vi "LMS_GetLPFBWRange.vi"(8 "error in (no error)":errorcluster, 10 "dir_tx":u8, 11 "device_In":i64) -> (0 "error out":errorcluster, 1 "range":cluster{"min":dbl, "max":dbl, "step":dbl}, 3 "device_Out":i64)   [LabVIEW 2018, in "LMS_LV_Drv.lvlib"]
uses:
  LMS_LV_Drv.lvlib
  C:/Program Files/PothosSDR/bin/LimeSuite.dll
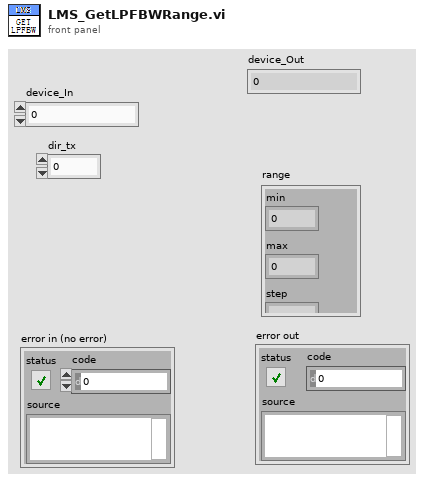
[diagram p1: front panel]
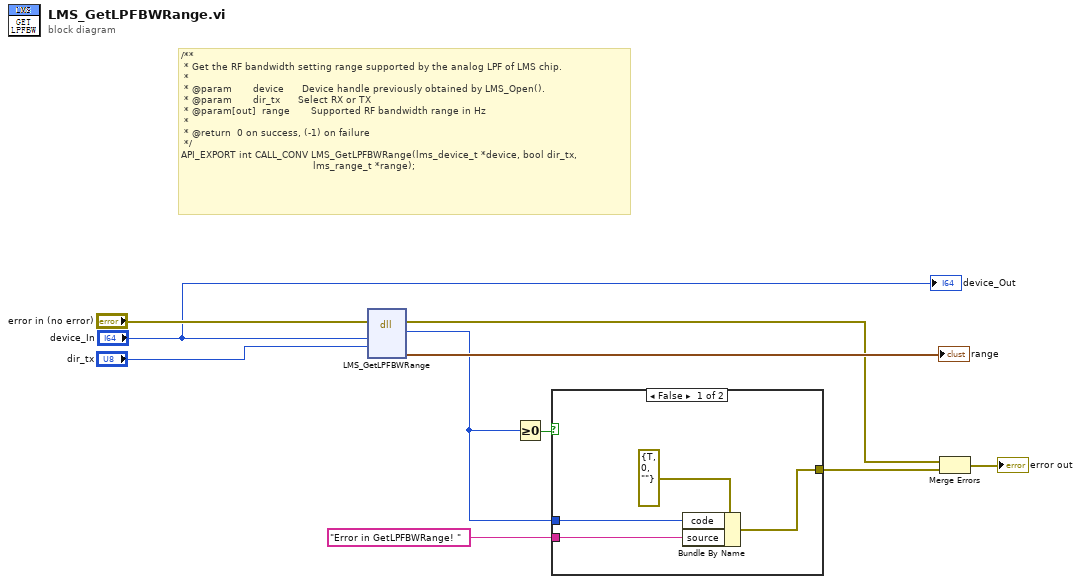
[diagram p0: block diagram]
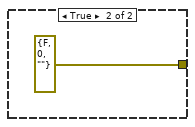
[diagram p2: hidden frame]
diagram:
  # "/**\n * Get the RF bandwidth setting range supported by the analog LPF of LMS chip.\n *\n * @param       device      Device handle previously obtained by LMS_Open().\n * @param       dir_tx      Select RX or TX\n * @param[out]  range       Supported RF bandwidth range in Hz\n *\n * @return  0 on success, (-1) on failure\n */\nAPI_EXPORT int CALL_CONV LMS_GetLPFBWRange(lms_device_t *device, bool dir_tx,\n                                            lms_range_t *range);"
  n1 = dll-call lib="C:/Program Files/PothosSDR/bin/LimeSuite.dll" fn="LMS_GetLPFBWRange"(error in="error in (no error)", "device"="device_In", "dir_tx"="dir_tx") -> (error out=w2:errorcluster, "return type"=w3:i32, "range"=→"range":cluster{"min":dbl, "max":dbl, "step":dbl})  [unwired: 5 in, 1 out]
  n2 = Greater Or Equal To 0?(x=w3) -> (x >= 0?=w6:bool)
  n3 = case shown="False" w6 {
    tunnel: [w13 errorcluster {"status"=FALSE, "code"=0, "source"=""} ("error in")] -> w4
    tunnel: w3 -> [w12 _]
    tunnel: "Error in GetLPFBWRange! " ("source") -> [w11 _]
    frame False {
      n4 = Bundle By Name(cluster=errorcluster {"status"=TRUE, "code"=0, "source"=""} ("error in"), "code"=w12, "source"=w11) -> (w13:errorcluster)
    }
    frame True {
    }
  }
  n5 = Merge Errors(w2, w4) -> (→"error out":errorcluster)
  "device_Out" <- "device_In"
